vi "FXPtoDAC.vi"(2 "Offset":i16, 3 "FXP In":fxp<+/-,16,12> format="%.30g") -> (0 "In Range?":bool, 1 "Coerced U16 Out":u16)   [LabVIEW 2011]
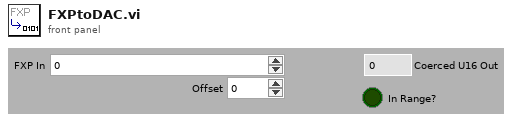
[diagram p1: front panel]
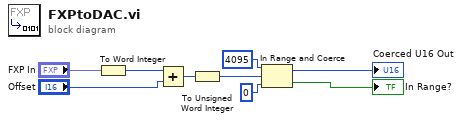
[diagram p0: block diagram]
diagram:
  n1 = To Word Integer(number="FXP In") -> (16bit integer=w7:i16)
  n2 = Add(x=w7, y="Offset") -> (x+y=w8:i16)
  n3 = To Unsigned Word Integer(number=w8) -> (unsigned 16bit integer=w9:u16)
  n4 = In Range and Coerce(upper limit=u16 4095, x=w9, lower limit=u16 0) -> (coerced(x)=→"Coerced U16 Out":u16, In Range?=→"In Range?":bool)
